vi "SMO Base Test Launcher.vi"() -> ()   [LabVIEW 2021, in "smo.lvlib"]
uses:
  smo.lvlib
  SMO.lvclass
  SMO.lvclass/SMO.ctl
  Typedefs/SMOState --Enum.ctl
  Private/ReftoDVR--SMO.vi
panel:
  out "error out":errorcluster
  # "Close Panel to stop the SMO\n(press the \"X\")"
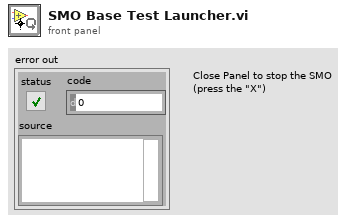
[diagram p1: front panel]
types:
  T1 = typedef "smo.lvlib/SMO.lvclass/Public Events.ctl" = cluster{"Error":refnum<user-event>, "State":refnum<user-event>, "Reserve State":refnum<user-event>}
  T2 = cluster{"Event Registration Refnum":refnum<event-registration>}
  T3 = typedef "smo.lvlib/SMO.lvclass/SMOState --Enum.ctl" = enum16{"unknown", "Created", "Started", "Stopped"}
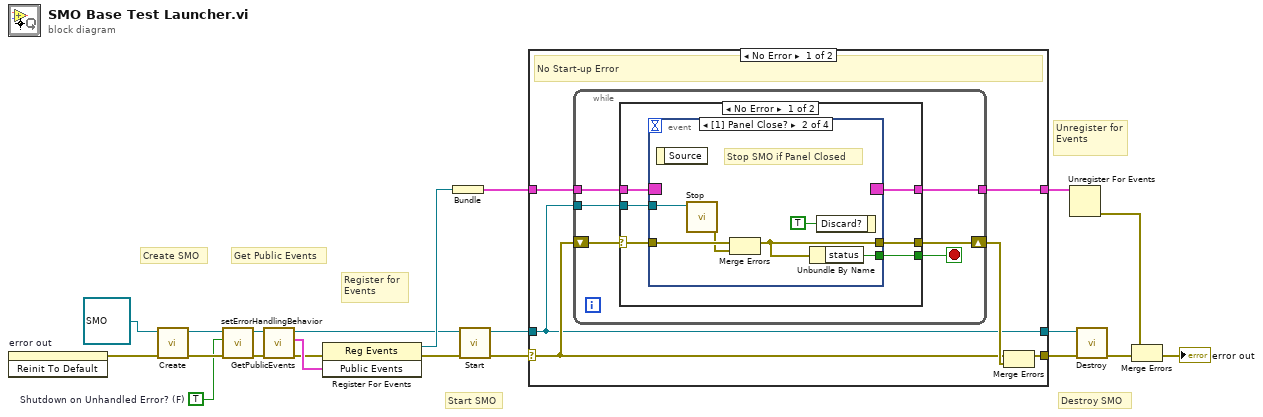
[diagram p0: block diagram]
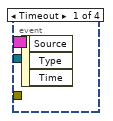
[diagram p2: hidden frame]
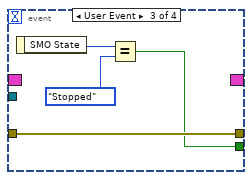
[diagram p3: hidden frame]
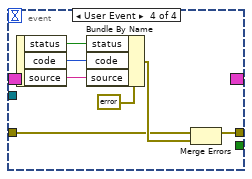
[diagram p4: hidden frame]
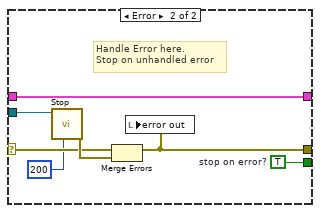
[diagram p5: hidden frame]
diagram:
  w6 = TRUE  # Shutdown on Unhandled Error? (F)
  # "Get Public Events"
  # "Start SMO"
  # "Destroy SMO"
  # "Create SMO"
  # "Unregister for Events"
  # "Register for Events"
  n1 = invoke on="error out" class="Clust (strict)" method="Reinit To Default"() -> (error out=w5:errorcluster)  [unwired: 3 in, 2 out]
  n2 = call "Create.vi"("error in (no error)"=w5, "SMO"=refnum<class "SMO.lvclass"> refnum) -> ("error out"=w8:errorcluster, "SMO out"=w10:refnum<class "SMO.lvclass">)  [unwired: 7 in, 1 out]
  n3 = call "setErrorHandlingBehavior.vi"("error in (no error)"=w8, "Shutdown on Unhandled Error? (F)"=w6, "SMO in"=w10) -> ("error out"=w7:errorcluster, "SMO out"=w9:refnum<class "SMO.lvclass">)  [unwired: 7 in]
  n4 = call "GetPublicEvents.vi"("error in (no error)"=w7, "SMO"=w9) -> ("error out"=w13:errorcluster, "Public Events"=w14:T1, "SMO out"=w4:refnum<class "SMO.lvclass">)  [unwired: 7 in]
  n5 = register-events(error in=w13, w14) -> (reference out=w16:refnum<event-registration>, error out=w15:errorcluster)  [unwired: 1 in]
  n6 = Bundle("Event Registration Refnum"=w16) -> (w20:T2)  [unwired: 1 in]
  n7 = call "Start.vi"("error in (no error)"=w15, "SMO"=w4) -> ("error out"=w2:errorcluster, "SMO out"=w3:refnum<class "SMO.lvclass">)  [unwired: 8 in]
  n8 = case shown="No Error" w2 {
    selector: w2 -> [w23 w65]
    tunnel: [w27 w66] -> w21
    tunnel: w20 -> [w26 w66]
    tunnel: [w24 w65] -> w12
    tunnel: w3 -> [w22 w64]
    tunnel: [w22 w64] -> w1
    frame No Error {
      # "No Start-up Error"
      n9 = while {
        shift-right: [w32] -> w25
        shift-left: w23 -> [w28]
        tunnel: w26 -> [w31]
        tunnel: [w30] -> w27
        tunnel: w22 -> [w29]
        stop <- w33 stop-if-true
        n10 = case shown="No Error" w28 {
          selector: w28 -> [w34 w60]
          tunnel: [w39 w63] -> w33
          tunnel: [w38 w57] -> w32
          tunnel: w31 -> [w37 w62]
          tunnel: [w36 w62] -> w30
          tunnel: w29 -> [w35 w59]
          frame No Error {
            n11 = event shown="[1] Panel Close?" {
              selector: w37 -> [_ _ _ _]
              dyn-events: [_ _ _ _] -> w36
              timeout: _ -> [_ _ _ _]
              tunnel: [_ w43 w46 _] -> w39
              tunnel: w35 -> [_ w45 _ _]
              tunnel: [_ w40 w47 w50] -> w38
              tunnel: w34 -> [_ w42 w47 w51]
              event Timeout {
                n12 = event-data() -> ()  [unwired: 1 in, 3 out]
              }
              event Panel Close? {
                # "Stop SMO if Panel Closed"
                n13 = event-data() -> ()  [unwired: 1 in, 1 out]
                n14 = call "Stop.vi"("SMO"=w45) -> ("error out"=w41:errorcluster)  [unwired: 9 in, 1 out]
                n15 = Merge Errors(w42, w41) -> (w40:errorcluster)
                n16 = Unbundle By Name(w40) -> ("status"=w43:bool)
                n17 = event-data("Discard?"=TRUE ("OK")) -> ()  [unwired: 1 in, 1 out]
              }
              event User Event {
                n18 = event-data() -> ("SMO State"=w49:T3)  [unwired: 1 in]
                n19 = Equal?(x=w49, y=SMOState_--Enum."Stopped") -> (x = y?=w46:bool)
              }
              event User Event {
                n20 = event-data() -> ("status"=w56:bool, "code"=w55:i32, "source"=w54:string)  [unwired: 1 in]
                n21 = Bundle By Name(cluster=errorcluster {"status"=FALSE, "code"=0, "source"=""} ("error out"), "status"=w56, "code"=w55, "source"=w54) -> (w52:errorcluster)
                n22 = Merge Errors(w51, w52) -> (w50:errorcluster)
              }
            }
          }
          frame Error {
            w63 = TRUE  # stop on error?
            # "Handle Error here.\nStop on unhandled error"
            n23 = call "Stop.vi"("timeout in ms (-1)"=200, "SMO"=w59) -> ("error out"=w61:errorcluster)  [unwired: 8 in, 1 out]
            n24 = Merge Errors(w60, w61) -> (w57:errorcluster)
            n25 = local write "error out"(w57) -> ()
          }
        }
      }
      n26 = Merge Errors(w23, w25) -> (w24:errorcluster)
    }
    frame Error {
      # "Error occured before starting the process"
    }
  }
  n27 = Unregister For Events(event registration refnum=w21) -> (error out=w19:errorcluster)  [unwired: 1 in]
  n28 = call "Destroy.vi"("error in (no error)"=w12, "SMO"=w1) -> ("error out"=w17:errorcluster)  [unwired: 9 in]
  n29 = Merge Errors(w19, w17) -> (→"error out":errorcluster)
